vi "Fetch Multi Eval Meas Spectrum Results.vi"(0 "VISA resource name":refnum<visa-resource-name>, 5 "Instance (1)":i32=1, 7 "Result Type (Current)":i32(ring) items=["Current"=0, "Maximum"=4], 11 "error in (no error)":errorcluster) -> (4 "VISA resource name out":refnum<visa-resource-name>, 6 "Reliability":i32, 8 "Results":dbl[](array[numeric]) format="%^.3e", 14 "Out Of Tolerance":dbl format="%^.3e", 15 "error out":errorcluster)   [LabVIEW 2015, in "Rohde&Schwarz CMP LR WPAN Measurement.lvlib"]
doc: "Returns the spectrum single results.\n\nAttribute:\n-\n\nRemote-control commands:\nFETCh:WPAN:MEAS<i>:MEValuation:SPECtrum:CURRent?\nFETCh:WPAN:MEAS<i>:MEValuation:SPECtrum:MAXimum?"
uses:
  <instrlib>/Rohde&Schwarz CMP LR WPAN Measurement/Rohde&Schwarz CMP LR WPAN Measurement.lvlib
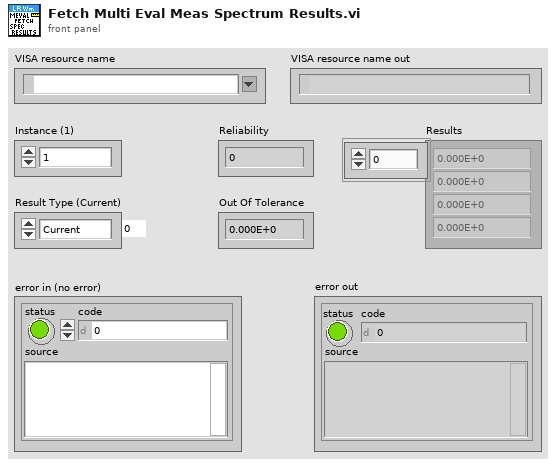
[diagram p1: front panel]
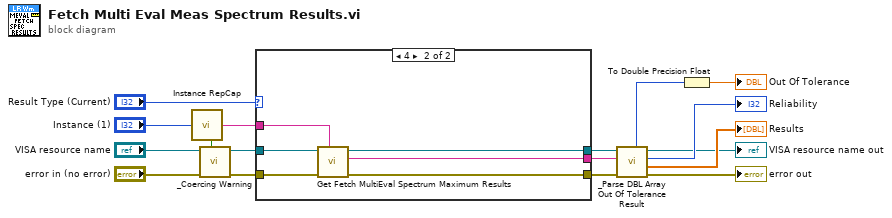
[diagram p0: block diagram]
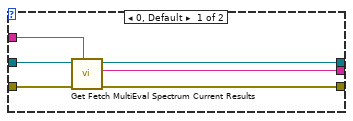
[diagram p2: hidden frame]
diagram:
  n1 = call <instrlib>:"Instance RepCap.vi"("Instance In"="Instance (1)") -> ("In Range?"=w16:bool, "RepCap Identifier Out"=w17:string)  [unwired: 1 in]
  n2 = call <instrlib>:"_Coercing Warning.vi"("In Range?"=w16, "error in (no error)"="error in (no error)", "VISA resource name"="VISA resource name") -> ("error out"=w13:errorcluster, "VISA resource name out"=w12:refnum<visa-resource-name>)  [unwired: 7 in]
  n3 = case shown="4" "Result Type (Current)" {
    tunnel: w17 -> [w23 w29]
    tunnel: w12 -> [w21 w27]
    tunnel: w13 -> [w22 w28]
    tunnel: [w18 w24] -> w4
    tunnel: [w20 w26] -> w3
    tunnel: [w19 w25] -> w2
    frame 0, Default {
      n4 = call "Get Fetch MultiEval Spectrum Current Results"("Repeated Capabilities"=w23, "error in (no error)"=w22, "instrument handle"=w21) -> ("error out"=w18:errorcluster, "Fetch MultiEval Spectrum Current Results"=w19:string, "instrument handle out"=w20:refnum<visa-resource-name>)  [unwired: 6 in]
    }
    frame 4 {
      n5 = call "Get Fetch MultiEval Spectrum Maximum Results"("Repeated Capabilities"=w29, "error in (no error)"=w28, "instrument handle"=w27) -> ("error out"=w24:errorcluster, "Fetch MultiEval Spectrum Maximum Results"=w25:string, "instrument handle out"=w26:refnum<visa-resource-name>)  [unwired: 6 in]
    }
  }
  n6 = call <instrlib>:"_Parse DBL Array Out Of Tolerance Result.vi"("error in (no error)"=w4, "Input String"=w2, "VISA resource name"=w3) -> ("error out"=→"error out":errorcluster, "Results"=→"Results":dbl[], "Reliability"=→"Reliability":i32, "VISA resource name out"=→"VISA resource name out":refnum<visa-resource-name>, "Out Of Tolerance"=w9:i32)  [unwired: 4 in]
  n7 = To Double Precision Float(number=w9) -> (double precision float=→"Out Of Tolerance":dbl)
